vi "Read Lockin Digitizer Driver.vi"(8 "error in (no error)":errorcluster, 11 "Lockin Digitizer in":refnum<class "Lockin Digitizer.lvclass">) -> (0 "error out":errorcluster, 2 "Lockin Digitizer Driver.lvclass":refnum<class "Lockin Digitizer Driver.lvclass">, 3 "Lockin Digitizer out":refnum<class "Lockin Digitizer.lvclass">)   [LabVIEW 2021, in "Lockin Digitizer.lvclass"]
uses:
  Lockin Digitizer.lvclass
  Lockin Digitizer.lvclass/Lockin Digitizer.ctl
  NHMFL_Core/Libraries/Instruments/Pulse Driver/Lockin Digitizer Driver/Lockin Digitizer Driver.lvclass
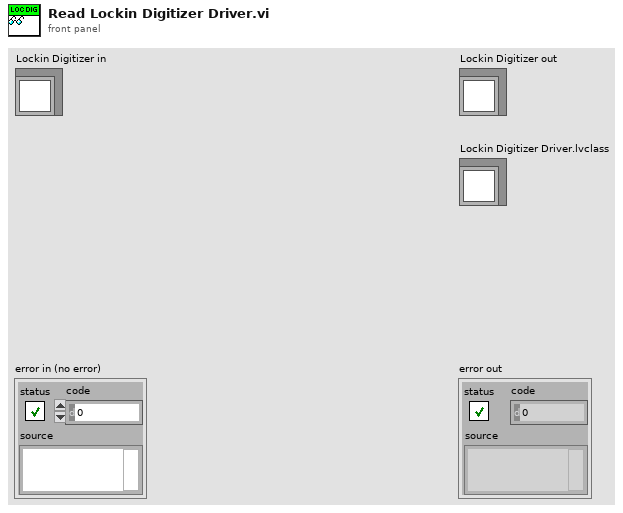
[diagram p1: front panel]
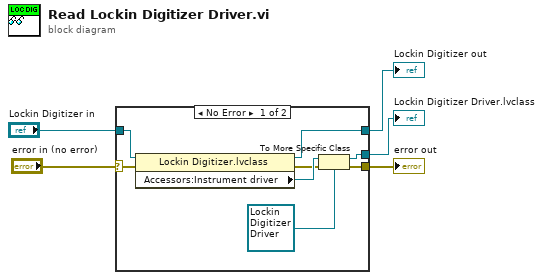
[diagram p0: block diagram]
diagram:
  n1 = case shown="No Error" "error in (no error)" {
    selector: "error in (no error)" -> [w13 w14]
    tunnel: [w7 w14] -> w4
    tunnel: [w11 w15] -> w2
    tunnel: "Lockin Digitizer in" -> [w12 w15]
    tunnel: [w6 _] -> w1
    frame No Error {
      n2 = property class="Lockin Digitizer.lvclass"(reference=w12, error in=w13) -> (reference out=w11:refnum<class "Lockin Digitizer.lvclass">, error out=w8:errorcluster, "Accessors:Instrument driver"=w9:refnum<class "Instrument Driver.lvclass">)
      n3 = To More Specific Class(target class=refnum<class "Lockin Digitizer Driver.lvclass"> refnum ("Lockin Digitizer Driver"), reference=w9, error in=w8) -> (specific class reference=w6:refnum<class "Lockin Digitizer Driver.lvclass">, error out=w7:errorcluster)
    }
    frame Error {
    }
  }
  "error out" <- w4
  "Lockin Digitizer out" <- w2
  "Lockin Digitizer Driver.lvclass" <- w1
